vi "Configure Sub-Sampling.vi"(7 "Sub-Sampling Source(1:Level)":u16(ring)=1 items=["External", "Level"], 8 "error in (no error)":errorcluster, 9 "Sample Interval (20E-6 s)":dbl=2e-05 format="%#.6g", 10 "Sample Count (1024)":dbl=1024.0 format="%#.6g", 11 "VISA resource name":refnum<visa-resource-name>) -> (0 "error out":errorcluster, 3 "VISA resource name out":refnum<visa-resource-name>)   [LabVIEW 2020, in "3458A Basic Driver.lvlib"]
doc: "Configures the DMM to start taking measurements using the sub-sampling method."
uses:
  3458A Basic Driver.lvlib
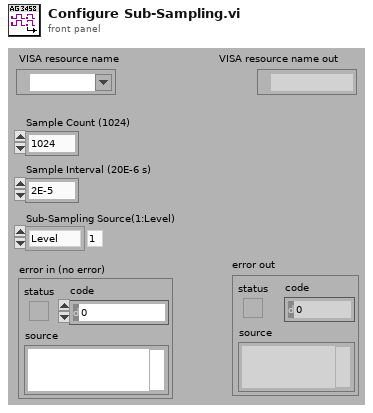
[diagram p1: front panel]
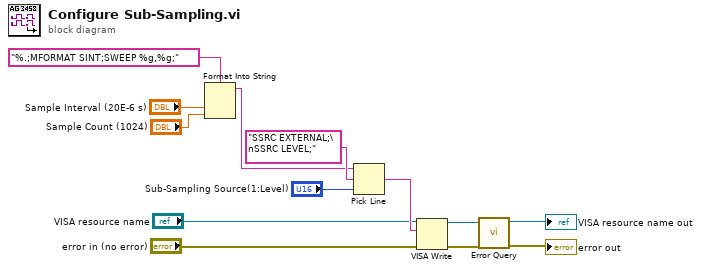
[diagram p0: block diagram]
diagram:
  n1 = Format Into String(format string="%.;MFORMAT SINT;SWEEP %g,%g;", "Sample Interval (20E-6 s)", "Sample Count (1024)") -> (resulting string=w8:string)  [unwired: 2 in, 1 out]
  n2 = Pick Line(string ("")=w8, multi-line string="SSRC EXTERNAL;\nSSRC LEVEL;", line index="Sub-Sampling Source(1:Level)") -> (output string=w7:string)
  n3 = VISA Write(VISA resource name="VISA resource name", write buffer=w7, error in (no error)="error in (no error)") -> (VISA resource name out=w5:refnum<visa-resource-name>, error out=w4:errorcluster)  [unwired: 1 out]
  n4 = call "Error Query.vi"("error in (no error)"=w4, "VISA resource name"=w5) -> ("error out"=→"error out":errorcluster, "VISA resource name out"=→"VISA resource name out":refnum<visa-resource-name>)  [unwired: 6 in, 2 out]
